vi "Hitech_init.vi"(8 "errin":errorcluster, 11 "VISA HITECH":string) -> (0 "error out":errorcluster, 3 "VisaHitech":refnum<visa-resource-name>)   [LabVIEW 2020]
uses:
  <instrlib>/IT6000C/IT6000C.lvlib
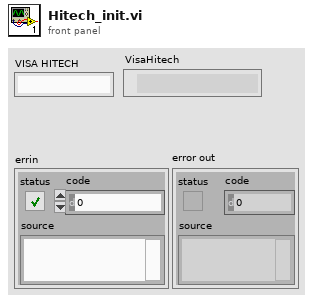
[diagram p1: front panel]
types:
  T1 = cluster{"Baud Rate":u32, "Parity":u16, "Data Bits":u16, "Stop Bits":u16, "Flow Control":u16}
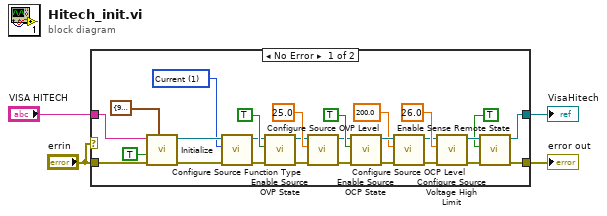
[diagram p0: block diagram]
diagram:
  n1 = case shown="No Error" "errin" {
    tunnel: "errin" -> [w31 w33]
    tunnel: "VISA HITECH" -> [w30 w32]
    tunnel: [w13 w32] -> w3
    tunnel: [w7 w33] -> w2
    frame No Error {
      w8 = u16 1 items=["Voltage", "Current"] ("Mode(0:Voltage)")
      n2 = call <instrlib>:"Initialize.vi"("Serial Configuration"=T1 {"Baud Rate"=9600, "Parity"=0, "Data Bits"=8, "Stop Bits"=10, "Flow Control"=0}, "error in (no error)"=w31, "Reset (True)"=TRUE, "VISA resource name"=w30) -> ("error out"=w12:errorcluster, "VISA resource name out"=w9:refnum<visa-resource-name>)  [unwired: 6 in]
      n3 = call <instrlib>:"Configure Source Function Type.vi"("error in (no error)"=w12, "Mode(0:Voltage)"=w8, "VISA resource name"=w9) -> ("error out"=w11:errorcluster, "VISA resource name out"=w10:refnum<visa-resource-name>)  [unwired: 7 in]
      n4 = call <instrlib>:"Enable Source OVP State.vi"("error in (no error)"=w11, "Enable(True)"=TRUE, "VISA resource name"=w10) -> ("error out"=w21:errorcluster, "VISA resource name out"=w19:refnum<visa-resource-name>)  [unwired: 7 in]
      n5 = call <instrlib>:"Configure Source OVP Level.vi"("error in (no error)"=w21, "Value(0)"=25.0, "VISA resource name"=w19) -> ("error out"=w17:errorcluster, "VISA resource name out"=w18:refnum<visa-resource-name>)  [unwired: 7 in]
      n6 = call <instrlib>:"Enable Source OCP State.vi"("error in (no error)"=w17, "Enable(True)"=TRUE, "VISA resource name"=w18) -> ("error out"=w27:errorcluster, "VISA resource name out"=w26:refnum<visa-resource-name>)  [unwired: 7 in]
      n7 = call <instrlib>:"Configure Source OCP Level.vi"("error in (no error)"=w27, "Value(0)"=200.0, "VISA resource name"=w26) -> ("error out"=w24:errorcluster, "VISA resource name out"=w22:refnum<visa-resource-name>)  [unwired: 7 in]
      n8 = call <instrlib>:"Configure Source Voltage High Limit.vi"("error in (no error)"=w24, "Value(0)"=26.0, "VISA resource name"=w22) -> ("error out"=w15:errorcluster, "VISA resource name out"=w16:refnum<visa-resource-name>)  [unwired: 7 in]
      n9 = call <instrlib>:"Enable Sense Remote State.vi"("error in (no error)"=w15, "Enable(True)"=TRUE, "VISA resource name"=w16) -> ("error out"=w7:errorcluster, "VISA resource name out"=w13:refnum<visa-resource-name>)  [unwired: 7 in]
    }
    frame Error {
    }
  }
  "VisaHitech" <- w3
  "error out" <- w2
